vi "Console_Run.vi"(10 "Code":string, 11 "Queue in":refnum<queue>) -> ()   [LabVIEW 2022 SP3]
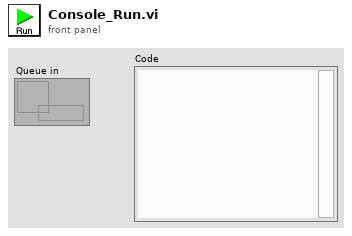
[diagram p1: front panel]
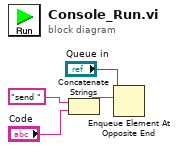
[diagram p0: block diagram]
diagram:
  n1 = Concatenate Strings("send " ("element"), "Code") -> (w2:string)
  n2 = Enqueue Element At Opposite End(queue="Queue in", element=w2) -> ()  [unwired: 2 in, 3 out]
